vi "PH_Revolver-GUI_6P.panel.vi"(0 "object ref":refnum<vi>, 5 "error in (no error)":errorcluster) -> (19 "error out":errorcluster)   [LabVIEW 2014, in "PH_Revolver-GUI_6P.lvlib"]
doc: "By this VI a ross relais can be monitored and switched. \n\nThe indicators \"CLOSED\", \"OPEN\" and \"SWITCH STATE\" show the value of the Beckhoff-Tag: blue indicates bad tag status reference problems, darkgreen false and lightgreen on. If everything is working fine, \"CLOSED\" and \"SWITCH STATE\" should show the same value, while \"OPEN\" has the opposite value. \n\nThe oval button switches the ross relais. It should be in the same state as the \"SWITCH STATE\" indicator. \n\n\"EXIT\" closes the front panel (GUI), while \"Delete Instance\" disconnects and removes the instance from the PCS.\n\nThis VI has no machine safety relevant logig: there is neither a check of internal conclict nor with other objects, for example conflict with other ross relais. Therefore it must be handled with care and should be operated by well educated operators only. It is forseen exclusively for direct operating and testing of the system. \n\nLicense Agreement for this software:\n\nCopyright (C)\nGesellschaft für Schwerionenforschung, GSI\nPlanckstr. 1\n64291 Darmstadt\nGermany\n\nContact: D.Beck@gsi.de \n\nThis program is free software; you can redistribute it and/or modify it under the terms of the GNU General Public License as published by the Free Software Foundation; either version 2 of the license, or (at your option) any later version.\n\nThis program is distributed in the hope that it will be useful, but WITHOUT ANYW ARRANTY; without even the implied warranty of MERCHANTABILITY or FITNESS FOR A PARTICULAR PURPOSE. See the GNU General License for more details (http://www.gnu.org).\n\nGesellschaft für Schwerionenforschung, GSI\nPlanckstr. 1, 64291 Darmstadt, Germany\nFor all questions and ideas contact: M.Richter@gsi.de, H.Brand@gsi.de or D.Beck@gsi.de.\nLast update: 18-DEC-2002"
uses:
  PH_Revolver-GUI_6P.lvlib
  PH_Basics/PH_Stepmotor_BaseClass/PH_Stepmotor_BaseClass.Axis Settings.ctl
  PH_Basics/PH_Stepmotor_BaseClass/PH_Stepmotor_BaseClass.Motor Type.ctl
  PH_Basics/PH_Stepmotor_BaseClass/PH_Stepmotor_BaseClass.Axis Address.ctl
  PH_Basics/PH_Stepmotor_BaseClass/PH_Stepmotor_BaseClass.Axis Activity.ctl
  PH_Basics/PH_AxisGUI_BaseClass/PH_AxisGUI_BaseClass.Axis GUI Refs.ctl
  PH_Basics/PH_Stepmotor_BaseClass/PH_Stepmotor_BaseClass.Axis Direction.ctl
  PH_Revolver-GUI_6P.Position.ctl
  CS_Core/CSObj/CSObj.lvlib
  PH_Basics/PH_Common/PH_Common.lvlib
  CS_Core/CSSystem/CSSystemLib/CSSystemLib.lvlib
  PH_Basics/PH_AxisGUI_BaseClass/PH_AxisGUI_BaseClass.lvlib
  PH_Basics/PH_Stepmotor_BaseClass/PH_Stepmotor_BaseClass.lvlib
  PH_Basics/PH_PSDBWriter/PH_PSDBWriter.lvlib
  PH_Basics/PH_Class/PH_Class.lvlib
panel:
  out "Status Bar":u32(colorbox)=16777088 caption="Axis1"
  out "Activity":T1
  out "Status":u32(colorbox)=6618880 caption="Axis1"
  in  "StopMotor":bool caption="SetZero"
  out "PSDB Status":u32(colorbox)=6618880 caption="PSDB"
  in  "Tab Control":enum32{"Move", "Settings", "Info"}(tab)
  in  "60°":bool
  in  "300°":bool
  in  "240°":bool
  in  "180°":bool
  in  "120°":bool
  in  "0°":bool
  out "Action":bool
  in  "DOWN":bool caption="? Steps"
  in  "UP":bool caption="? Steps"
  in  "Axis_Target":string="0" caption="Steps"
  in  "Clear Error":bool
  in  "Axis_Settings":T2={"Sign change"=FALSE, "Width"=0.0, "Calibration"=0.0, "Unit"="Steps", "Motor Type"=enum."Unspecific", "Unit Width"="", "Unit CF"=""} caption="Axis"
  in  "Reset":bool
  out "Address":T4={"Instance"="N/A", "Motor Nr"=0} caption="Sixpack"
  in  "Set Zero":bool
  in  "Delete":bool
  in  "Exit":bool
  # "PCS"
  # "3.40"
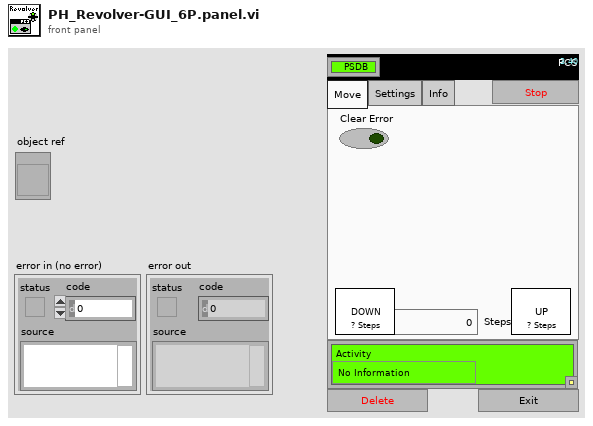
[diagram p1: front panel]
types:
  T1 = typedef "PH_Stepmotor_BaseClass.lvlib/PH_Stepmotor_BaseClass.Axis Activity.ctl" = enum16{"No Information", "stopped", "running", "Failure", "Alarm", "stopped at backward ES", "stopped at foreward ES"}
  T2 = typedef "PH_Stepmotor_BaseClass.lvlib/PH_Stepmotor_BaseClass.Axis Settings.ctl" = cluster{"Sign change":bool, "Width":dbl, "Calibration":dbl, "Unit":string, "Motor Type":T3, "Unit Width":string, "Unit CF":string}
  T3 = typedef "PH_Stepmotor_BaseClass.lvlib/PH_Stepmotor_BaseClass.Motor Type.ctl" = enum16{"Unspecific", "OWIS 49.120.2633", "OWIS 49.060.1033", "OWIS 43.040.2558", "Diamond Motion 2200 series", "OWIS 49.120.266B.MV6", "Calorimeter", "Linear Stage 1", "MICOS VT-80", "MICOS VT-80 S", "Standa Rotstage nt0.95A", "PUF RA 320.200", "PUF RA 800.200", "PUF RA 800.400", "PUF RA 400.50", "1324.nn.800.50", "1324.n9c.800.50", "1324.nn.320.200", "1324.nn.400.200", "1324.nn.800.200", "1324.nn.400.50", "1324.8c9c.800.50", "1324.8c9c.400.200"}
  T4 = typedef "PH_Stepmotor_BaseClass.lvlib/PH_Stepmotor_BaseClass.Axis Address.ctl" = cluster{"Instance":string, "Motor Nr":i32}
  T5 = typedef "PH_AxisGUI_BaseClass.lvlib/PH_AxisGUI_BaseClass.Axis GUI Refs.ctl" = cluster{"Back":refnum<vi>, "Forth":refnum<vi>, "Status":refnum<vi>, "Target":refnum<vi>, "Address":refnum<vi>, "Status Bar":refnum<vi>, "Settings":refnum<vi>, "Activity":refnum<vi>, "Clear Error":refnum<vi>}
  T6 = typedef "PH_Stepmotor_BaseClass.lvlib/PH_Stepmotor_BaseClass.Axis Direction.ctl" = enum16{"forward", "backward"}
  T7 = typedef "PH_Revolver-GUI_6P.lvlib/PH_Revolver-GUI_6P.Position.ctl" = u16
  T8 = typedef "PH_AxisGUI_BaseClass.lvlib/PH_AxisGUI_BaseClass.i attribute.ctl" = cluster{"Axes":T9[]}
  T9 = typedef "PH_AxisGUI_BaseClass.lvlib/PH_AxisGUI_BaseClass.Axis Attributes.ctl" = cluster{"Axis GUI Refs":T5, "Address":T4, "Name":string, "Label \"Back\"":string, "Labell \"Forth\"":string, "Moving?":bool}
  T10 = typedef "PH_Revolver-GUI_6P.lvlib/PH_Revolver-GUI_6P.i attribute.ctl" = cluster{"GUI Refs":cluster{"0°":refnum<vi>, "60°":refnum<vi>, "120°":refnum<vi>, "180°":refnum<vi>, "240°":refnum<vi>, "300°":refnum<vi>, "Action":refnum<vi>}, "Revolver Position":T7, "Service ID Position":i32, "Captions":string[]}
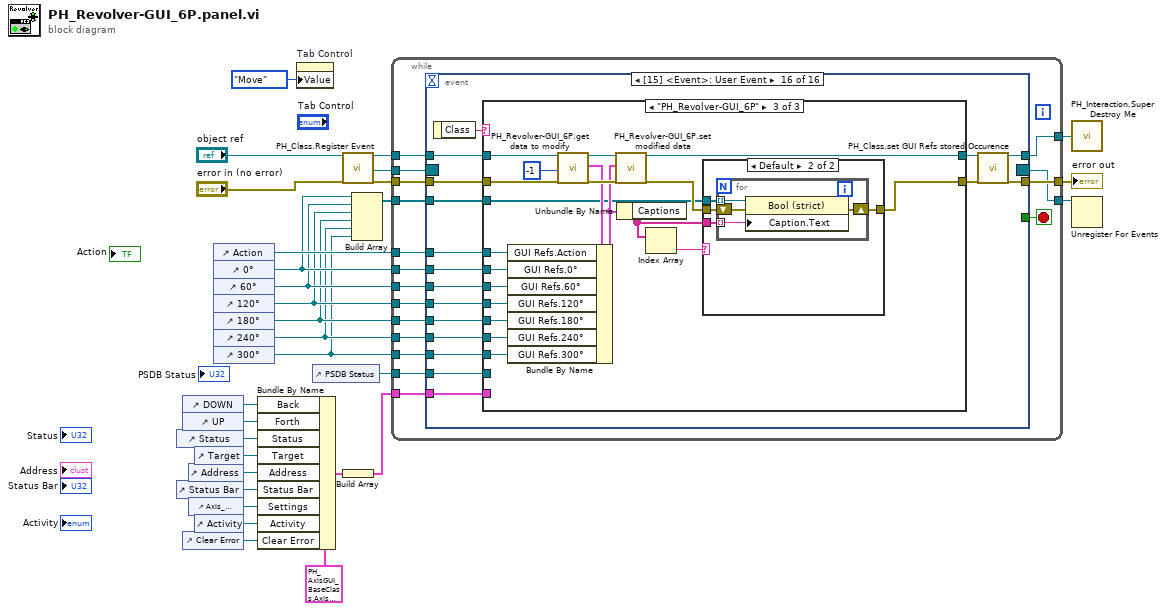
[diagram p0: block diagram]
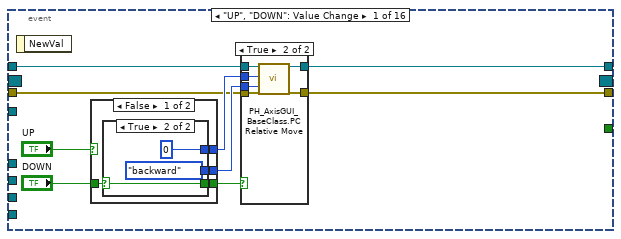
[diagram p2: hidden frame]
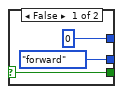
[diagram p3: hidden frame]
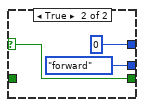
[diagram p4: hidden frame]
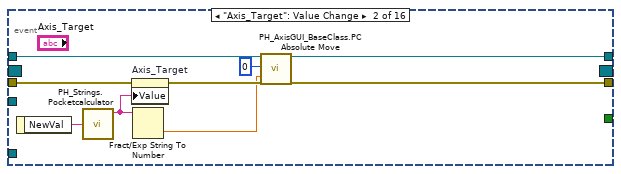
[diagram p6: hidden frame]
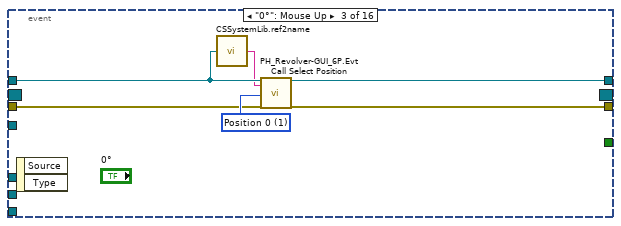
[diagram p7: hidden frame]
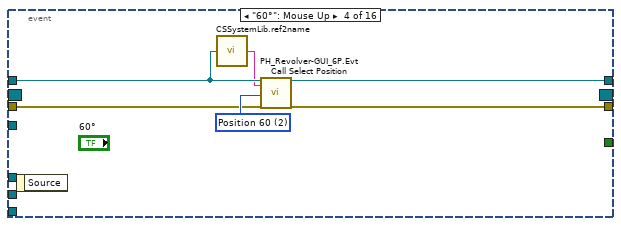
[diagram p8: hidden frame]
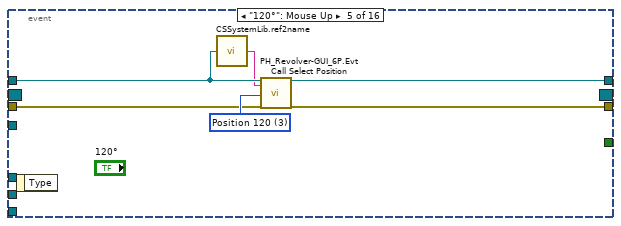
[diagram p9: hidden frame]
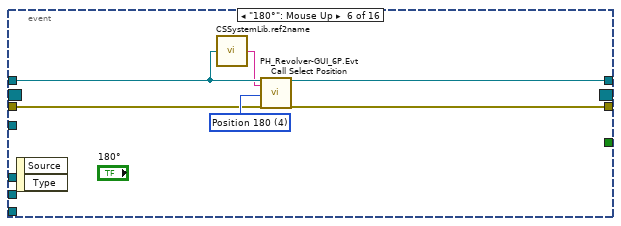
[diagram p10: hidden frame]
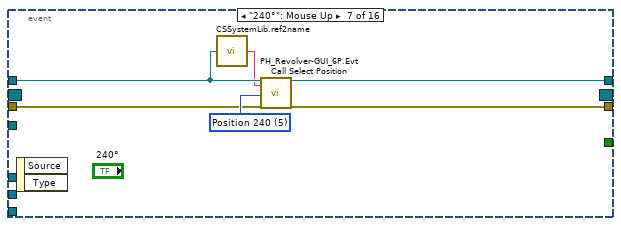
[diagram p11: hidden frame]
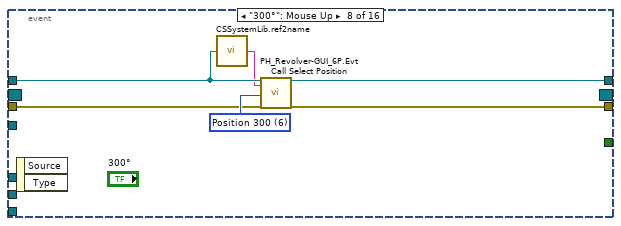
[diagram p12: hidden frame]
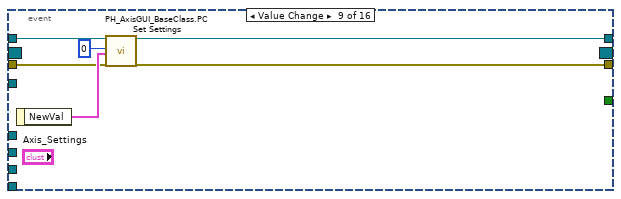
[diagram p13: hidden frame]
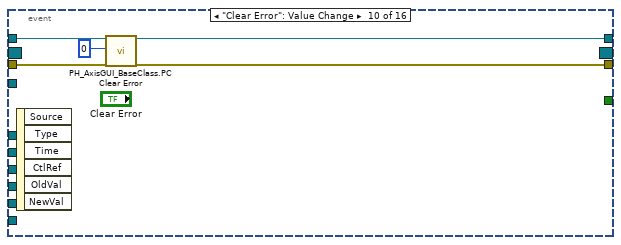
[diagram p14: hidden frame]
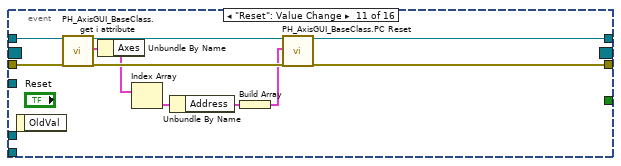
[diagram p15: hidden frame]
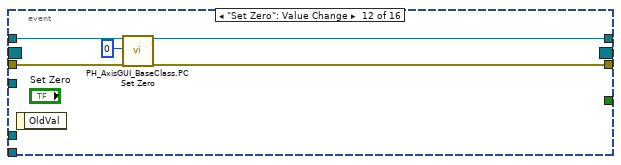
[diagram p16: hidden frame]
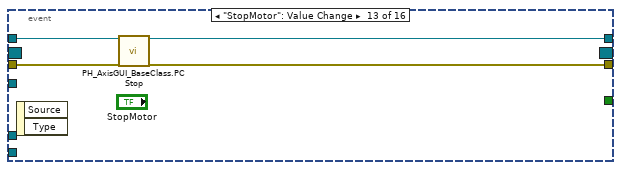
[diagram p17: hidden frame]
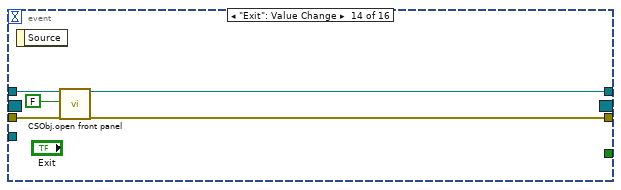
[diagram p18: hidden frame]
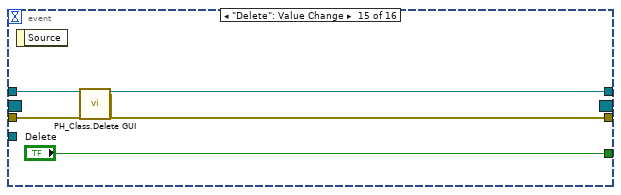
[diagram p19: hidden frame]
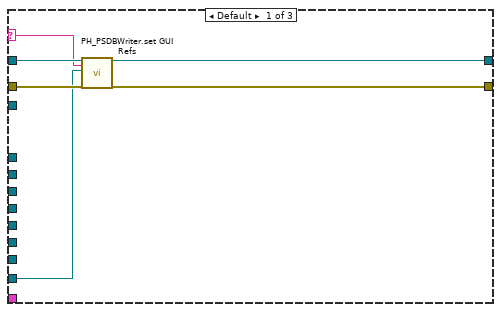
[diagram p20: hidden frame]
diagram:
  n1 = control-ref of="Status"() -> (w18:refnum<vi>)
  n2 = control-ref of="Status Bar"() -> (w19:refnum<vi>)
  n3 = control-ref of="DOWN"() -> (w22:refnum<vi>)
  n4 = control-ref of="UP"() -> (w23:refnum<vi>)
  n5 = control-ref of="Clear Error"() -> (w17:refnum<vi>)
  n6 = control-ref of="Address"() -> (w24:refnum<vi>)
  n7 = control-ref of="Axis_Settings"() -> (w21:refnum<vi>)
  n8 = control-ref of="Target"() -> (w25:refnum<vi>)
  n9 = control-ref of="Activity"() -> (w20:refnum<vi>)
  n10 = control-ref of="Action"() -> (w11:refnum<vi>)
  n11 = control-ref of="0°"() -> (w10:refnum<vi>)
  n12 = control-ref of="60°"() -> (w9:refnum<vi>)
  n13 = control-ref of="120°"() -> (w8:refnum<vi>)
  n14 = control-ref of="180°"() -> (w7:refnum<vi>)
  n15 = control-ref of="240°"() -> (w6:refnum<vi>)
  n16 = control-ref of="300°"() -> (w5:refnum<vi>)
  n17 = Bundle By Name(cluster=T5 {"Back"=refnum, "Forth"=refnum, "Status"=refnum, "Target"=refnum, "Address"=refnum, "Status Bar"=refnum, "Settings"=refnum, "Activity"=refnum, "Clear Error"=refnum} ("GUI Refs"), "Back"=w22, "Forth"=w23, "Status"=w18, "Target"=w25, "Address"=w24, "Status Bar"=w19, "Settings"=w21, "Activity"=w20, "Clear Error"=w17) -> (w26:T5)
  n18 = property on="Tab Control" class="TabCtl (strict)"("Value"=enum32{"Move", "Settings", "Info"}."Move" ("Tab Control")) -> ()  [unwired: 2 in, 2 out]
  n19 = control-ref of="PSDB Status"() -> (w13:refnum<vi>)
  n20 = call "PH_Class.Register Event.vi"("i ref in"="object ref", "error in (no error)"="error in (no error)") -> ("i ref out"=w16:refnum<vi>, "Event Registration Refnum"=w14:refnum<event-registration>, "error out"=w15:errorcluster)  [unwired: 15 in]
  n21 = Build Array(w26) -> (w12:T5[])
  n22 = Build Array(w10, w9, w8, w7, w6, w5) -> (w1:refnum<vi>[])
  n23 = while {
    tunnel: w16 -> [w44]
    tunnel: [w43] -> w29
    tunnel: w15 -> [w46]
    tunnel: [w45] -> w30
    tunnel: w14 -> [w42]
    tunnel: w13 -> [w41]
    tunnel: w12 -> [w40]
    tunnel: w11 -> [w39]
    tunnel: w10 -> [w38]
    tunnel: w9 -> [w37]
    tunnel: w8 -> [w36]
    tunnel: w7 -> [w35]
    tunnel: w6 -> [w34]
    tunnel: w5 -> [w33]
    tunnel: [w32] -> w4
    tunnel: w1 -> [w31]
    stop <- w47 stop-if-true
    n24 = event shown="[15] <Event>: User Event" {
      selector: w42 -> [_ _ _ _ _ _ _ _ _ _ _ _ _ _ _ _]
      dyn-events: [_ _ _ _ _ _ _ _ _ _ _ _ _ _ _ _] -> w32
      timeout: _ -> [_ _ _ _ _ _ _ _ _ _ _ _ _ _ _ _]
      tunnel: [_ _ _ _ _ _ _ _ _ _ _ _ _ _ "Delete" _] -> w47
      tunnel: w44 -> [w49 w80 w89 w95 w101 w107 w113 w119 w125 w131 w142 w147 w151 w158 w162 w180]
      tunnel: w46 -> [w48 w79 w87 w93 w99 w105 w111 w117 w124 w130 w141 w146 w150 w156 w161 w179]
      tunnel: [w51 w85 w92 w98 w104 w110 w116 w122 w128 w133 w144 w149 w152 w155 w159 w167] -> w45
      tunnel: [w50 w84 w91 w97 w103 w109 w115 w121 w127 w132 w143 w148 w153 w154 w160 w165] -> w43
      tunnel: w41 -> [_ _ _ _ _ _ _ _ _ _ _ _ _ _ _ w177]
      tunnel: w40 -> [_ _ _ _ _ _ _ _ _ _ _ _ _ _ _ w175]
      tunnel: w39 -> [_ _ _ _ _ _ _ _ _ _ _ _ _ _ _ w174]
      tunnel: w38 -> [_ _ _ _ _ _ _ _ _ _ _ _ _ _ _ w173]
      tunnel: w37 -> [_ _ _ _ _ _ _ _ _ _ _ _ _ _ _ w172]
      tunnel: w36 -> [_ _ _ _ _ _ _ _ _ _ _ _ _ _ _ w171]
      tunnel: w35 -> [_ _ _ _ _ _ _ _ _ _ _ _ _ _ _ w170]
      tunnel: w34 -> [_ _ _ _ _ _ _ _ _ _ _ _ _ _ _ w169]
      tunnel: w33 -> [_ _ _ _ _ _ _ _ _ _ _ _ _ _ _ w168]
      tunnel: w31 -> [_ _ _ _ _ _ _ _ _ _ _ _ _ _ _ w164]
      event "UP", "DOWN": Value Change {
        n25 = event-data() -> ()  [unwired: 1 in, 1 out]
        n26 = case shown="False" "UP" {
          selector: "UP" -> [_ w67]
          tunnel: [w60 0] -> w55
          tunnel: [w59 PH_Stepmotor_BaseClass.Axis_Direction."forward" ("direction")] -> w56
          tunnel: "DOWN" -> [w58 _]
          tunnel: [w57 w67] -> w54
          frame False {
            n27 = case shown="True" w58 {
              selector: w58 -> [w61 w64]
              tunnel: [0 0] -> w60
              tunnel: [PH_Stepmotor_BaseClass.Axis_Direction."forward" ("direction") PH_Stepmotor_BaseClass.Axis_Direction."backward" ("direction")] -> w59
              tunnel: [w61 w64] -> w57
              frame False {
              }
              frame True {
              }
            }
          }
          frame True {
          }
        }
        n28 = case shown="True" w54 {
          tunnel: w48 -> [w70 w77]
          tunnel: w49 -> [w71 w76]
          tunnel: w56 -> [_ w75]
          tunnel: [w71 w74] -> w50
          tunnel: [w70 w73] -> w51
          tunnel: w55 -> [_ w72]
          frame False {
          }
          frame True {
            n29 = call "PH_AxisGUI_BaseClass.PC Relative Move.vi"("i ref in"=w76, "Axis"=w72, "direction"=w75, "error in"=w77) -> ("i ref out"=w74:refnum<vi>, "error out"=w73:errorcluster)  [unwired: 14 in]
          }
        }
      }
      event "Axis_Target": Value Change {
        n30 = event-data() -> ("NewVal"=w86:string)  [unwired: 1 in]
        n31 = call "PH_Strings.Pocketcalculator.vi"("Input"=w86) -> ("String Double"=w83:string)  [unwired: 3 out]
        n32 = property on="Axis_Target" class="Str"(error in=w79, "Value"=w83) -> (error out=w82:errorcluster)  [unwired: 1 in, 1 out]
        n33 = Fract/Exp String To Number(string=w83) -> (number=w81:dbl)  [unwired: 3 in, 1 out]
        n34 = call "PH_AxisGUI_BaseClass.PC Absolute Move.vi"("i ref in"=w80, "Axis"=0, "Position [Units]"=w81, "error in"=w82) -> ("i ref out"=w84:refnum<vi>, "error out"=w85:errorcluster)  [unwired: 14 in]
      }
      event "0°": Mouse Up {
        w90 = T7 1 items=["unknown", "Position 0", "Position 60", "Position 120", "Position 180", "Position 240", "Position 300", "moving"] ("Wanted Position")
        n35 = event-data() -> ()  [unwired: 1 in, 2 out]
        n36 = call "CSSystemLib.ref2name.vi"("obj refnum"=w89) -> ("name"=w88:string)
        n37 = call "PH_Revolver-GUI_6P.Evt Call Select Position.vi"("i ref in"=w89, "Revolver Instance"=w88, "Wanted Position"=w90, "error in"=w87) -> ("i ref out"=w91:refnum<vi>, "error out"=w92:errorcluster)  [unwired: 14 in]
      }
      event "60°": Mouse Up {
        w96 = T7 2 items=["unknown", "Position 0", "Position 60", "Position 120", "Position 180", "Position 240", "Position 300", "moving"] ("Wanted Position")
        n38 = event-data() -> ()  [unwired: 1 in, 1 out]
        n39 = call "CSSystemLib.ref2name.vi"("obj refnum"=w95) -> ("name"=w94:string)
        n40 = call "PH_Revolver-GUI_6P.Evt Call Select Position.vi"("i ref in"=w95, "Revolver Instance"=w94, "Wanted Position"=w96, "error in"=w93) -> ("i ref out"=w97:refnum<vi>, "error out"=w98:errorcluster)  [unwired: 14 in]
      }
      event "120°": Mouse Up {
        w102 = T7 3 items=["unknown", "Position 0", "Position 60", "Position 120", "Position 180", "Position 240", "Position 300", "moving"] ("Wanted Position")
        n41 = event-data() -> ()  [unwired: 1 in, 1 out]
        n42 = call "CSSystemLib.ref2name.vi"("obj refnum"=w101) -> ("name"=w100:string)
        n43 = call "PH_Revolver-GUI_6P.Evt Call Select Position.vi"("i ref in"=w101, "Revolver Instance"=w100, "Wanted Position"=w102, "error in"=w99) -> ("i ref out"=w103:refnum<vi>, "error out"=w104:errorcluster)  [unwired: 14 in]
      }
      event "180°": Mouse Up {
        w108 = T7 4 items=["unknown", "Position 0", "Position 60", "Position 120", "Position 180", "Position 240", "Position 300", "moving"] ("Wanted Position")
        n44 = event-data() -> ()  [unwired: 1 in, 2 out]
        n45 = call "CSSystemLib.ref2name.vi"("obj refnum"=w107) -> ("name"=w106:string)
        n46 = call "PH_Revolver-GUI_6P.Evt Call Select Position.vi"("i ref in"=w107, "Revolver Instance"=w106, "Wanted Position"=w108, "error in"=w105) -> ("i ref out"=w109:refnum<vi>, "error out"=w110:errorcluster)  [unwired: 14 in]
      }
      event "240°": Mouse Up {
        w114 = T7 5 items=["unknown", "Position 0", "Position 60", "Position 120", "Position 180", "Position 240", "Position 300", "moving"] ("Wanted Position")
        n47 = event-data() -> ()  [unwired: 1 in, 2 out]
        n48 = call "CSSystemLib.ref2name.vi"("obj refnum"=w113) -> ("name"=w112:string)
        n49 = call "PH_Revolver-GUI_6P.Evt Call Select Position.vi"("i ref in"=w113, "Revolver Instance"=w112, "Wanted Position"=w114, "error in"=w111) -> ("i ref out"=w115:refnum<vi>, "error out"=w116:errorcluster)  [unwired: 14 in]
      }
      event "300°": Mouse Up {
        w120 = T7 6 items=["unknown", "Position 0", "Position 60", "Position 120", "Position 180", "Position 240", "Position 300", "moving"] ("Wanted Position")
        n50 = event-data() -> ()  [unwired: 1 in, 2 out]
        n51 = call "CSSystemLib.ref2name.vi"("obj refnum"=w119) -> ("name"=w118:string)
        n52 = call "PH_Revolver-GUI_6P.Evt Call Select Position.vi"("i ref in"=w119, "Revolver Instance"=w118, "Wanted Position"=w120, "error in"=w117) -> ("i ref out"=w121:refnum<vi>, "error out"=w122:errorcluster)  [unwired: 14 in]
      }
      event Value Change {
        n53 = event-data() -> ("NewVal"=w126:T2)  [unwired: 1 in]
        n54 = call "PH_AxisGUI_BaseClass.PC Set Settings.vi"("VI in"=w125, "Axis"=0, "NewVal"=w126, "error in (no error)"=w124) -> ("VI out"=w127:refnum<vi>, "error out"=w128:errorcluster)  [unwired: 14 in]
      }
      event "Clear Error": Value Change {
        n55 = event-data() -> ()  [unwired: 1 in, 6 out]
        n56 = call "PH_AxisGUI_BaseClass.PC Clear Error.vi"("i ref in"=w131, "Axis"=0, "error in"=w130) -> ("i ref out"=w132:refnum<vi>, "error out"=w133:errorcluster)  [unwired: 15 in]
      }
      event "Reset": Value Change {
        n57 = event-data() -> ()  [unwired: 1 in, 1 out]
        n58 = call "PH_AxisGUI_BaseClass.get i attribute.vi"("i ref in"=w142, "error in (no error)"=w141) -> ("i ref out"=w140:refnum<vi>, "i attribute"=w138:T8, "error out"=w139:errorcluster)  [unwired: 15 in]
        n59 = Unbundle By Name(w138) -> ("Axes"=w136:T9[])
        n60 = Index Array(array=w136) -> (element=w137:T9)  [unwired: 1 in]
        n61 = Unbundle By Name(w137) -> ("Address"=w135:T4)
        n62 = Build Array(w135) -> (w134:T4[])
        n63 = call "PH_AxisGUI_BaseClass.PC Reset.vi"("i ref in"=w140, "Addresses"=w134, "error in"=w139) -> ("i ref out"=w143:refnum<vi>, "error out"=w144:errorcluster)  [unwired: 15 in]
      }
      event "Set Zero": Value Change {
        n64 = event-data() -> ()  [unwired: 1 in, 1 out]
        n65 = call "PH_AxisGUI_BaseClass.PC Set Zero.vi"("VI in"=w147, "Axis"=0, "error in (no error)"=w146) -> ("VI out"=w148:refnum<vi>, "error out"=w149:errorcluster)  [unwired: 15 in]
      }
      event "StopMotor": Value Change {
        n66 = event-data() -> ()  [unwired: 1 in, 2 out]
        n67 = call "PH_AxisGUI_BaseClass.PC Stop.vi"("VI in"=w151, "error in (no error)"=w150) -> ("VI out"=w153:refnum<vi>, "error out"=w152:errorcluster)  [unwired: 16 in]
      }
      event "Exit": Value Change {
        n68 = event-data() -> ()  [unwired: 1 in, 1 out]
        n69 = call "CSObj.open front panel.vi"("i ref in"=w158, "frontPanelOpen"=FALSE ("front panel open"), "error in (no error)"=w156) -> ("i ref out"=w154:refnum<vi>, "error out"=w155:errorcluster)  [unwired: 15 in]
      }
      event "Delete": Value Change {
        n70 = event-data() -> ()  [unwired: 1 in, 1 out]
        n71 = call "PH_Class.Delete GUI.vi"("VI in"=w162, "error in (no error)"=w161) -> ("VI out"=w160:refnum<vi>, "error out"=w159:errorcluster)  [unwired: 16 in]
      }
      event User Event {
        n72 = event-data() -> ("Class"=w176:string)  [unwired: 1 in]
        n73 = case shown="\"PH_Revolver-GUI_6P\"" w176 {
          selector: w176 -> [w181 w188 _]
          tunnel: w180 -> [w186 w192 w208]
          tunnel: w179 -> [w185 w190 w207]
          tunnel: [w184 w189 w195] -> w178
          tunnel: [w183 w191 w206] -> w166
          tunnel: w177 -> [w182 _ _]
          tunnel: w175 -> [_ w187 _]
          tunnel: w174 -> [_ _ w205]
          tunnel: w173 -> [_ _ w204]
          tunnel: w172 -> [_ _ w203]
          tunnel: w171 -> [_ _ w202]
          tunnel: w170 -> [_ _ w201]
          tunnel: w169 -> [_ _ w200]
          tunnel: w168 -> [_ _ w199]
          tunnel: w164 -> [_ _ w193]
          frame Default {
            n74 = call "PH_PSDBWriter.set GUI Refs.vi"("i ref in"=w186, "Class"=w181, "Ref PSDB Status"=w182, "error in"=w185) -> ("i ref out"=w183:refnum<vi>, "error out"=w184:errorcluster)  [unwired: 14 in]
          }
          frame "PH_AxisGUI_BaseClass" {
            n75 = call "PH_AxisGUI_BaseClass.set GUI Refs.vi"("i ref in"=w192, "Class"=w188, "Axis GUI Base Class Refs"=w187, "error in"=w190) -> ("i ref out"=w191:refnum<vi>, "error out"=w189:errorcluster)  [unwired: 14 in]
          }
          frame "PH_Revolver-GUI_6P" {
            n76 = call "PH_Revolver-GUI_6P.get data to modify.vi"("i ref in"=w208, "ms timeout (10000)"=-1, "error in (no error)"=w207) -> ("i ref out"=w212:refnum<vi>, "i attribute"=w209:T10, "error out"=w211:errorcluster)  [unwired: 13 in, 1 out]
            n77 = Bundle By Name(cluster=w209, "GUI Refs.Action"=w205, "GUI Refs.0°"=w204, "GUI Refs.60°"=w203, "GUI Refs.120°"=w202, "GUI Refs.180°"=w201, "GUI Refs.240°"=w200, "GUI Refs.300°"=w199) -> (w198:T10)
            n78 = call "PH_Revolver-GUI_6P.set modified data.vi"("i ref in"=w212, "i attribute"=w198, "error in (no error)"=w211) -> ("i ref out"=w206:refnum<vi>, "error out"=w196:errorcluster)  [unwired: 15 in]
            n79 = Unbundle By Name(w198) -> ("Captions"=w197:string[])
            n80 = Index Array(array=w197) -> (element=w194:string)  [unwired: 1 in]
            n81 = case shown="Default" w194 {
              tunnel: w196 -> [w213 w217]
              tunnel: [w213 w216] -> w195
              tunnel: w193 -> [_ w215]
              tunnel: w197 -> [_ w214]
              frame "", "N/A" {
              }
              frame Default {
                n82 = for {
                  tunnel: w215 -> [w219] mode=indexing
                  shift-right: [w220] -> w216
                  shift-left: w217 -> [w221]
                  tunnel: w214 -> [w218] mode=indexing
                  n83 = property class="Bool (strict)"(reference=w219, error in=w221, "Caption.Text"=w218) -> (error out=w220:errorcluster)  [unwired: 1 out]
                }
              }
            }
          }
        }
        n84 = call "PH_Class.set GUI Refs stored Occurence.vi"("i ref in"=w166, "error in (no error)"=w178) -> ("i ref out"=w165:refnum<vi>, "error out"=w167:errorcluster)  [unwired: 16 in]
      }
    }
  }
  "error out" <- w30
  n85 = call "PH_Interaction.Super Destroy Me.vi"("i ref out"=w29) -> ()
  n86 = Unregister For Events(event registration refnum=w4) -> ()  [unwired: 1 in, 1 out]
